vi "Get Focus Index.vi"(8 "error in (no error)":errorcluster, 11 "Scalable Border in":refnum<class "Scalable Border.lvclass">) -> (0 "error out":errorcluster, 2 "Focus Index":i8, 3 "Scalable Border out":refnum<class "Scalable Border.lvclass">)   [LabVIEW 2015, in "Scalable Border.lvclass"]
uses:
  Scalable Border.lvclass
  Scalable Border.lvclass/Scalable Border.ctl
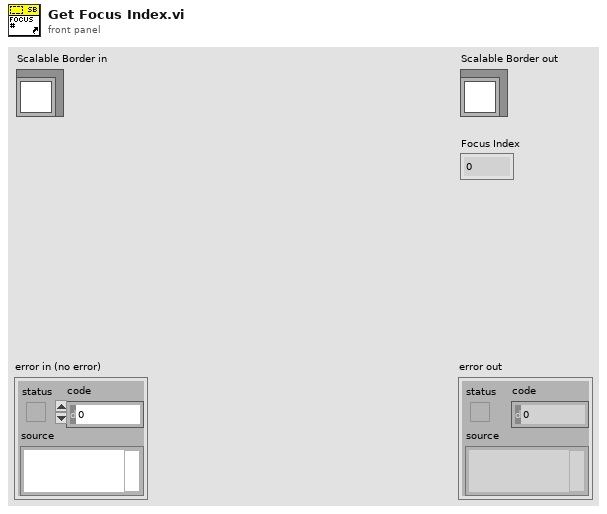
[diagram p1: front panel]
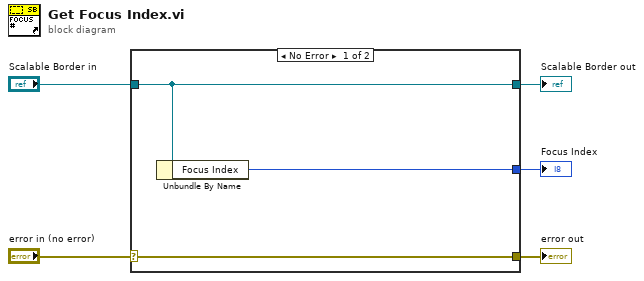
[diagram p0: block diagram]
diagram:
  n1 = case shown="No Error" "error in (no error)" {
    selector: "error in (no error)" -> [w8 w9]
    tunnel: [w8 w9] -> w4
    tunnel: [w7 w10] -> w2
    tunnel: "Scalable Border in" -> [w7 w10]
    tunnel: [w6 _] -> w1
    frame No Error {
      n2 = Unbundle By Name(w7) -> ("Focus Index"=w6:i8)
    }
    frame Error {
    }
  }
  "error out" <- w4
  "Scalable Border out" <- w2
  "Focus Index" <- w1
